vi "EEV Position.vi"() -> (3 "DSM Message":string)   [LabVIEW 2016]
uses:
  Custom Pallet Controls/Custom Pallet Forward.ctl
  LabVIEW GEA2 Toolkit v1.0.0.0/library/GEA2_Toolkit.lvlib
panel:
  in  "EEV Position":u16
  out "Description":string="Set EEV Position"
  in  "Complete":T1
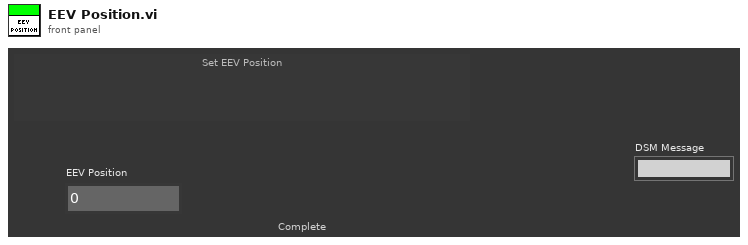
[diagram p1: front panel]
types:
  T1 = typedef "Custom Pallet Forward.ctl" = bool
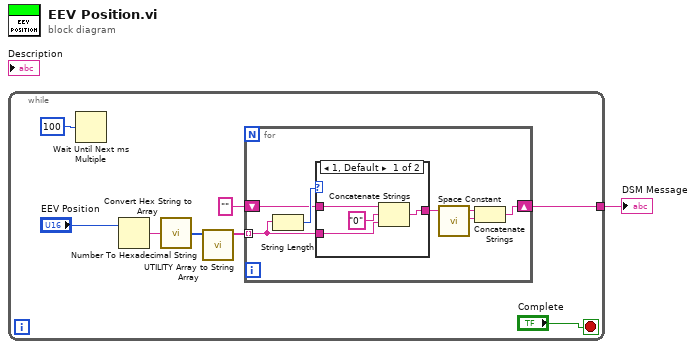
[diagram p0: block diagram]
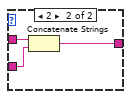
[diagram p2: hidden frame]
diagram:
  n1 = while {
    tunnel: [w4] -> w1
    stop <- "Complete" stop-if-true
    n2 = Wait Until Next ms Multiple(millisecond multiple=u32 100) -> ()  [unwired: 1 out]
    n3 = Number To Hexadecimal String(2:"EEV Position") -> (0:w6:string)  [unwired: 1 in]
    n4 = call "Convert Hex String to Array.vi"("Hex String In"=w6) -> ("Hex Array Out"=w3:u8[])  [unwired: 14 in]
    n5 = call "UTILITY Array to String Array.vi"("Hex Array Out"=w3) -> ("Array"=w2:string[])  [unwired: 9 in, 1 out]
    n6 = for {
      tunnel: w2 -> [w13] mode=indexing
      shift-right: [w10] -> w4
      shift-left: "" -> [w14]
      n7 = String Length(string=w13) -> (length=w15:i32)
      n8 = case shown="1, Default" w15 {
        tunnel: w14 -> [w19 w22]
        tunnel: [w16 w21] -> w11
        tunnel: w13 -> [w17 w20]
        frame 1, Default {
          n9 = Concatenate Strings(w19, "0" ("string"), w17) -> (w16:string)
        }
        frame 2 {
          n10 = Concatenate Strings(w22, w20) -> (w21:string)
        }
      }
      n11 = call <vilib>:"Space Constant.vi"() -> ("String"=w12:string)
      n12 = Concatenate Strings(w11, w12) -> (w10:string)
    }
  }
  "DSM Message" <- w1
